vi "Read Specs URL.vi"(8 "error in (no error)":errorcluster, 11 "VI Package in":refnum<class "VIPM Package.lvclass">) -> (0 "error out":errorcluster, 2 "Specs URL":string, 3 "VI Package out":refnum<class "VIPM Package.lvclass">)   [LabVIEW 2016, in "Packages.lvlib" / "VIPM Package.lvclass"]
uses:
  VIPM Package.lvclass
  VIPM Package.lvclass/VIPM Package.ctl
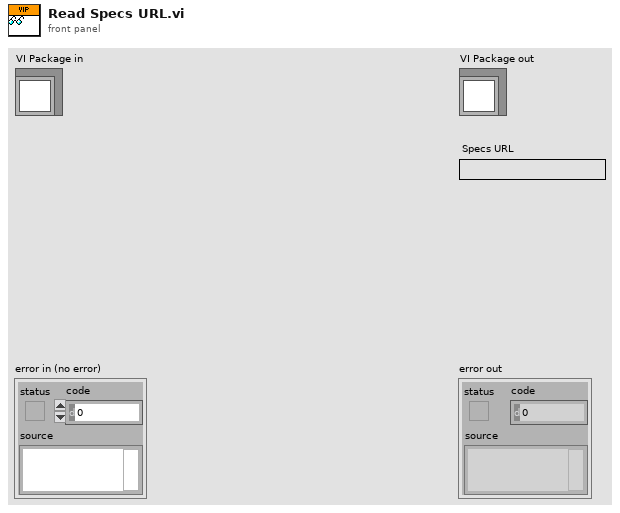
[diagram p1: front panel]
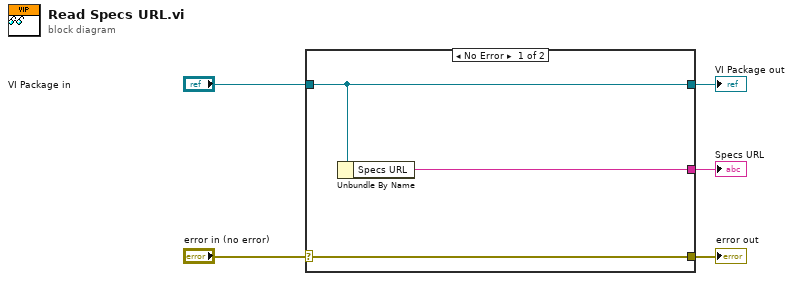
[diagram p0: block diagram]
diagram:
  n1 = case shown="No Error" "error in (no error)" {
    selector: "error in (no error)" -> [w8 w9]
    tunnel: [w8 w9] -> w4
    tunnel: [w7 w10] -> w2
    tunnel: "VI Package in" -> [w7 w10]
    tunnel: [w6 _] -> w1
    frame No Error {
      n2 = Unbundle By Name(w7) -> ("Specs URL"=w6:string)
    }
    frame Error {
    }
  }
  "error out" <- w4
  "VI Package out" <- w2
  "Specs URL" <- w1
